vi "Histogram.vi"(1 "Array in":u32[][](array[numeric])) -> (0 "Array out":dbl[][](array[numeric]))   [LabVIEW 2020]
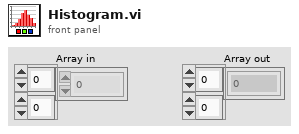
[diagram p1: front panel]
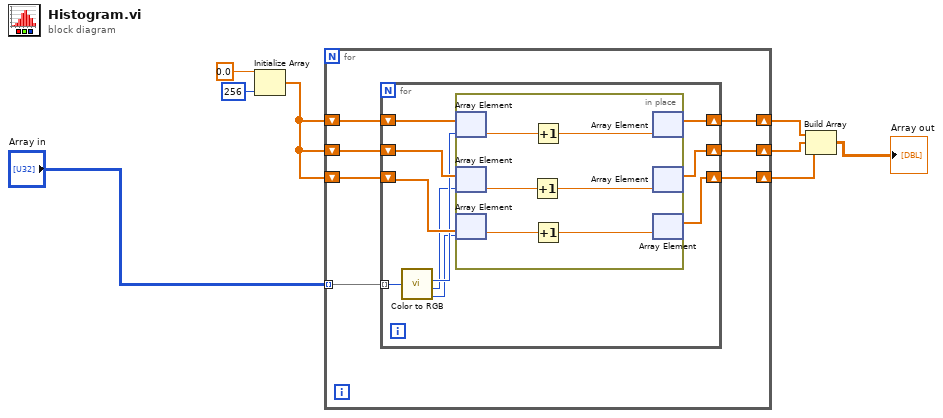
[diagram p0: block diagram]
diagram:
  n1 = Initialize Array(0.0 ("element"), 256 ("dimension size")) -> (w3:dbl[])
  n2 = for {
    shift-right: [w12] -> w5
    shift-left: w3 -> [w15]
    shift-right: [w11] -> w6
    shift-left: w3 -> [w14]
    shift-right: [w10] -> w7
    shift-left: w3 -> [w13]
    tunnel: "Array in" -> [w9] mode=indexing
    n3 = for {
      shift-right: [w18] -> w12
      shift-left: w15 -> [w25]
      shift-right: [w17] -> w11
      shift-left: w14 -> [w24]
      shift-right: [w16] -> w10
      shift-left: w13 -> [w23]
      tunnel: w9 -> [w22] mode=indexing
      n4 = call <vilib>:"Color to RGB.vi"("Color"=w22) -> ("R"=w21:u8, "G"=w20:u8, "B"=w19:u8)  [unwired: 1 out]
      n5 = in-place {
        n6 = in-place-array #1(w25, w21) -> (w26:dbl)
        n7 = in-place-array #2(w24, w20) -> (w29:dbl)
        n8 = in-place-array #3(w23, w19) -> (w28:dbl)
        n9 = Increment(x=w29) -> (x+1=w30:dbl)
        n10 = Increment(x=w26) -> (x+1=w31:dbl)
        n11 = Increment(x=w28) -> (x+1=w27:dbl)
        n12 = in-place-array #1(w31) -> (w18:dbl[])  [unwired: 1 out]
        n13 = in-place-array #2(w30) -> (w17:dbl[])  [unwired: 1 out]
        n14 = in-place-array #3(w27) -> (w16:dbl[])  [unwired: 1 out]
      }
    }
  }
  n15 = Build Array(w5, w6, w7) -> (→"Array out":dbl[][])
